vi "Parse Signature Algorithm.vi"(10 "error in (no error)":errorcluster, 11 "Header":string) -> (2 "error out":errorcluster, 3 "Signature Algorithm":T1)   [LabVIEW 2015, in "JWT.lvlib" / "JWT.lvclass"]
uses:
  JWT.lvclass
  Signature Algorithms.ctl
  JWT.lvlib
  lv-json/JSON/JSON.lvlib
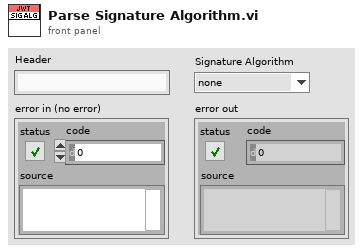
[diagram p1: front panel]
types:
  T1 = typedef "JWT.lvlib/Signature Algorithms.ctl" = enum16{"none", "HS256"}
  T2 = typedef "JSON.lvlib/JSON Item Type.ctl" = enum16{"unknown", "null", "Array", "Object", "String", "Number", "Boolean"}
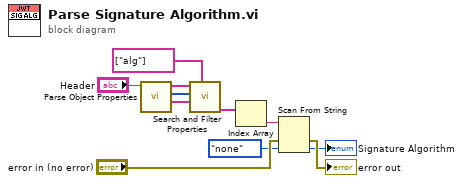
[diagram p0: block diagram]
diagram:
  n1 = call "Parse Object Properties.vi"("JSON String"="Header") -> ("Values"=w8:string[], "Item Types"=w9:T2[], "Keys"=w10:string[])  [unwired: 7 in, 1 out]
  n2 = call "Search and Filter Properties.vi"("Search Keys"=string[] ["alg"], "Values In"=w8, "Types In"=w9, "Keys In"=w10) -> ("Filtered Values"=w6:string[])  [unwired: 2 in, 5 out]
  n3 = Index Array(array=w6) -> (element=w4:string)  [unwired: 1 in]
  n4 = Scan From String(input string=w4, error in="error in (no error)", default 1=Signature_Algorithms."none" ("Signature Algorithms")) -> (error out=→"error out":errorcluster, output 1=→"Signature Algorithm":T1)  [unwired: 2 in, 2 out]
